vi "WaitOnListener.vi"(8 "error in (no error)":errorcluster, 11 "TCPIP in":refnum<class "TCPIP.lvclass">) -> (0 "error out":errorcluster, 3 "TCPIP out":refnum<class "TCPIP.lvclass">)   [LabVIEW 2018, in "TCPIP.lvclass"]
uses:
  TCPIP.lvclass
  TCPIP.lvclass/TCPIP.ctl
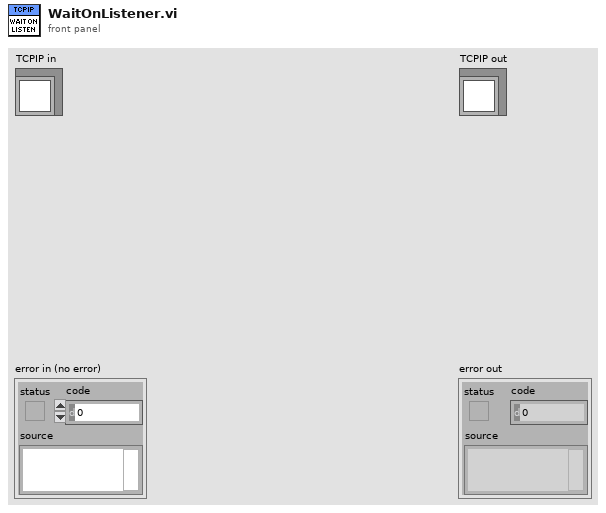
[diagram p1: front panel]
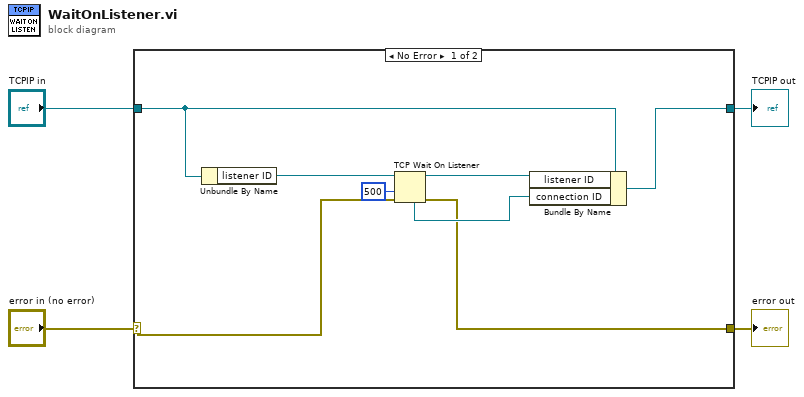
[diagram p0: block diagram]
diagram:
  n1 = case shown="No Error" "error in (no error)" {
    selector: "error in (no error)" -> [w6 w14]
    tunnel: [w5 w14] -> w3
    tunnel: [w10 w13] -> w1
    tunnel: "TCPIP in" -> [w11 w13]
    frame No Error {
      n2 = Unbundle By Name(w11) -> ("listener ID"=w12:refnum<k5>)
      n3 = TCP Wait On Listener(8:w6, 9:500 ("timeout ms (wait forever: -1)"), 11:w12) -> (0:w5:errorcluster, 3:w9:refnum<k5>, 4:w7:refnum<k5>)  [unwired: 1 in, 2 out]
      n4 = Bundle By Name(cluster=w11, "listener ID"=w9, "connection ID"=w7) -> (w10:refnum<class "TCPIP.lvclass">)
    }
    frame Error {
    }
  }
  "error out" <- w3
  "TCPIP out" <- w1
